vi "fxp32_to_i32.vi"(1 "fxp32_16":fxp<+/-,32,16>) -> (0 "32bit integer":i32)   [LabVIEW 2018]
uses:
  <vilib>/rvi/FXPMathLib/FxpInterpret/XNode/nifxpmath_Interpret.xnode
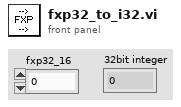
[diagram p1: front panel]
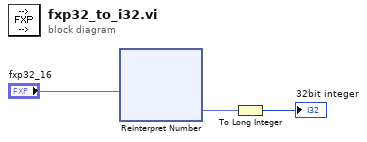
[diagram p0: block diagram]
diagram:
  n1 = xnode "Reinterpret Number"("x"="fxp32_16") -> ("y"=w2:fxp<+/-,32,32>)
  n2 = To Long Integer(number=w2) -> (32bit integer=→"32bit integer":i32)
